vi "User_Database_Close.vi"(8 "error in (no error)":errorcluster caption="错误输入（无错误）", 11 "SQLite Connection in":refnum<class "Connection.lvclass">) -> (0 "error out":errorcluster caption="错误输出")   [LabVIEW 2020]
uses:
  <vilib>/drjdpowell/SQLite Library/SQL Connection/Connection.lvclass
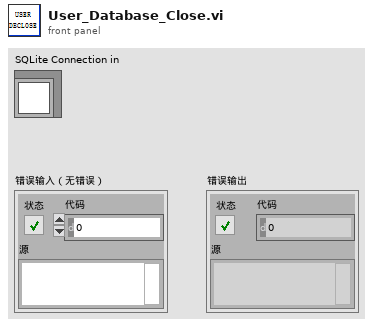
[diagram p1: front panel]
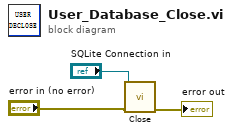
[diagram p0: block diagram]
diagram:
  n1 = call-dynamic "Close.vi"("error in (no error)"="error in (no error)", "SQLite Connection in"="SQLite Connection in") -> ("error out"=→"error out":errorcluster)  [unwired: 9 in]
